vi "DAQmx Task 2 Channels.vi"(11 "DAQmx Task Name":refnum<k21>) -> (3 "Channels Out":string[](array[string]))   [LabVIEW 2013]
uses:
  <resource>/objmgr/daqmx.rc
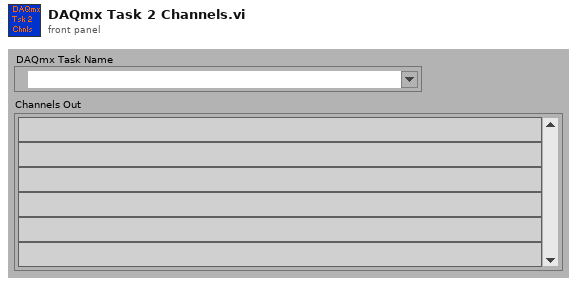
[diagram p1: front panel]
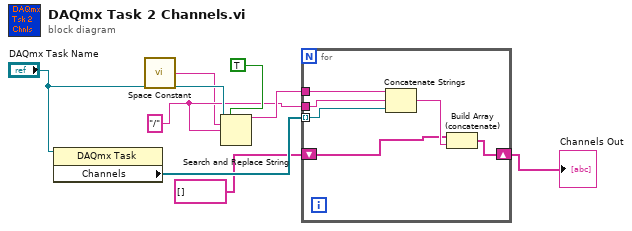
[diagram p0: block diagram]
diagram:
  w2 = "/"
  n1 = property class="DAQmx Task"(reference="DAQmx Task Name") -> ("Channels"=w5:refnum<k21>[])  [unwired: 1 in, 2 out]
  n2 = call <vilib>:"Space Constant.vi"() -> ("String"=w1:string)
  n3 = Search and Replace String(replace all?=TRUE ("replace all? (F)"), input string="DAQmx Task Name", search string=w1, replace string=w2) -> (result string=w6:string)  [unwired: 1 in, 6 out]
  n4 = for {
    shift-right: [w10] -> w4
    shift-left: string[] [] -> [w11]
    tunnel: w6 -> [w14]
    tunnel: w2 -> [w9]
    tunnel: w5 -> [w13] mode=indexing
    n5 = Concatenate Strings(w14, w9, w13) -> (w12:string)
    n6 = Build Array (concatenate)(w11, w12) -> (w10:string[])
  }
  "Channels Out" <- w4
